vi "zhemv - Hermitian Matrix-Vector Product (CDB).vi"(4 "beta":cdb=1.0+0.0i, 6 "alpha":cdb=1.0+0.0i, 8 "matrix A type":T1=3 items=["Lower Triangular"=2, "Upper Triangular"=3], 9 "y":cdb[](array[numeric]), 10 "x":cdb[](array[numeric]), 11 "A":T2) -> (0 "error":i32, 3 "zhemv":cdb[](array[numeric]))   [LabVIEW 2014, in "NI_AALBLAS.lvlib"]
doc: "Calculates the product of a Hermitian matrix and a vector."
uses:
  NI_AALBLAS.lvlib
  ComplexMatrix.ctl
  LV_UpLo.ctl
  Order.ctl
  Fucntion.ctl
  BLAS2 Utility(CDB).vi
  NI_Matrix.lvlib
panel:
  # "zhemv=alpha*A*x+beta*y"
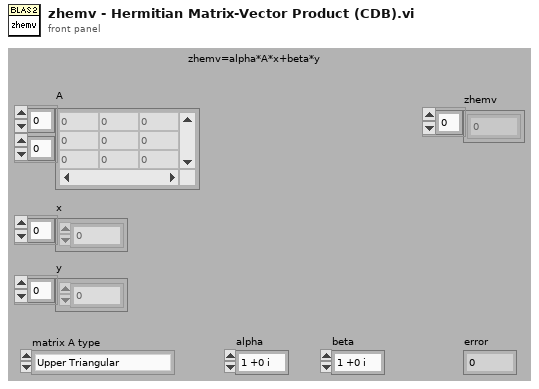
[diagram p1: front panel]
types:
  T1 = typedef "NI_AALBLAS.lvlib/LV_UpLo.ctl" = i32
  T2 = typedef "NI_Matrix.lvlib/ComplexMatrix.ctl" = cdb[][]
  T3 = typedef "NI_AALBLAS.lvlib/Fucntion.ctl" = u16
  T4 = typedef "NI_AALBLAS.lvlib/Order.ctl" = i32
  T5 = typedef "NI_AALBLAS.lvlib/UpLo.ctl" = i32
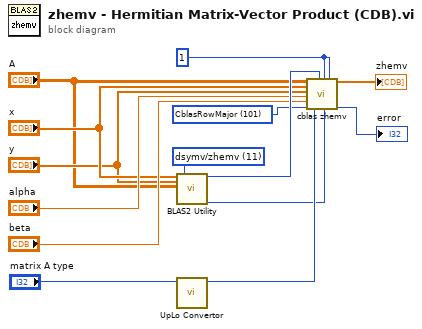
[diagram p0: block diagram]
diagram:
  w1 = T3 11 items=["ddot/zdotu/zdotc", "daxpy/zaxpy", "dnrm2/dznrm2", "dasum/dzasum", "dcopy/zcopy", "dswap/zswap", "drotm", "drot/zdrot", "idamax/izamax", "idamin/izamin", "dgemv/zgemv", "dsymv/zhemv", "dtrmv/ztrmv", "dsyr/zher", "dsyr2/zher2", "dger/zgeru/zgerc", "dtrsv/ztrsv", "dgemm/zgemm", "dsymm/zsymm/zhemm", "dtrmm/ztrmm", "dsyrk/zsyrk/zherk", "dsyr2k/zsyr2k/zher2k", "dtrsm/ztrsm"] ("function")
  w2 = T4 101 items=["CblasRowMajor"=101, "CblasColMajor"=102] ("order")
  w4 = 1
  n1 = call-poly "BLAS2 Utility.vi"("x"="x", "y"="y", "A"="A", "function"=w1) -> ("lda"=w14:i32, "n"=w3:i32)  [unwired: 1 in, 13 out]
  n2 = call "UpLo Convertor.vi"("triangle matrix type"="matrix A type") -> ("uplo"=w10:T5)  [unwired: 10 out]
  n3 = call "cblas zhemv.vi"("A"="A", "x"="x", "y"="y", "alpha"="alpha", "beta"="beta", "order"=w2, "uplo"=w10, "lda"=w14, "incx"=w4, "n"=w3, "incy"=w4) -> ("zhemv"=→"zhemv":cdb[], "error"=→"error":i32)  [unwired: 7 out]
